vi "源强计算.vi"() -> ()   [LabVIEW 2020]
uses:
  <vilib>/Analysis/6fits.llb/Curve Fitting Criteria.ctl
  <vilib>/Utility/inputDevices.llb/mouseAcquire.vi
  <vilib>/gmath/NumericalOptimization/Nonlinear Curve Fit LM.vi
  <vilib>/gmath/NI_Gmath.lvlib
  <vilib>/Analysis/NI_AALPro.lvlib
panel:
  in  "本底迭代步长":dbl[](array[numeric])=[0.0, 0.0, 0.0]
  in  "曲线显隐":bool[](array[boolean])
  in  "选项卡控件":enum32{"直线拟合(两参)", "混合多项式(三参)", "广指拟合(三参) "}(tab)
  in  "parameter bounds":T1={"slope min"=-inf, "slope max"=inf, "intercept min"=-inf, "intercept max"=inf} caption="参数界限"
  in  "初始参数":dbl[](array[numeric])
  in  "参数界限":T2={"amp min"=-inf, "amp max"=inf, "damping min"=-inf, "damping max"=inf, "offset min"=-inf, "offset max"=inf}
  in  "本底值":dbl[](array[numeric])=[0.0, 0.0, 0.0]
  out "两参法残差":dbl[](array[numeric])
  out "通量拟合源强":dbl[](array[numeric])
  out "两参法源强":dbl[](array[numeric])
  out "两参法反应性":dbl[](array[numeric])
  out "通量拟合残差":dbl[](array[numeric])
  in  "曲线标尺":bool[](array[boolean])
  in  "开始计算":bool
  in  "重选文件":bool
  in  "退出程序":bool
  out "提示信息":string
  out "filepath":path caption="数据文件路径和名称"
  out "数据采集起止时间":string
  out "DataGraph":dbl[][](graph)
  out "中间标位置":i32
  out "左选标位置":i32
  out "右选标位置":i32
  # "y=aX + b"
  # "y = a*exp(b*x) + c"
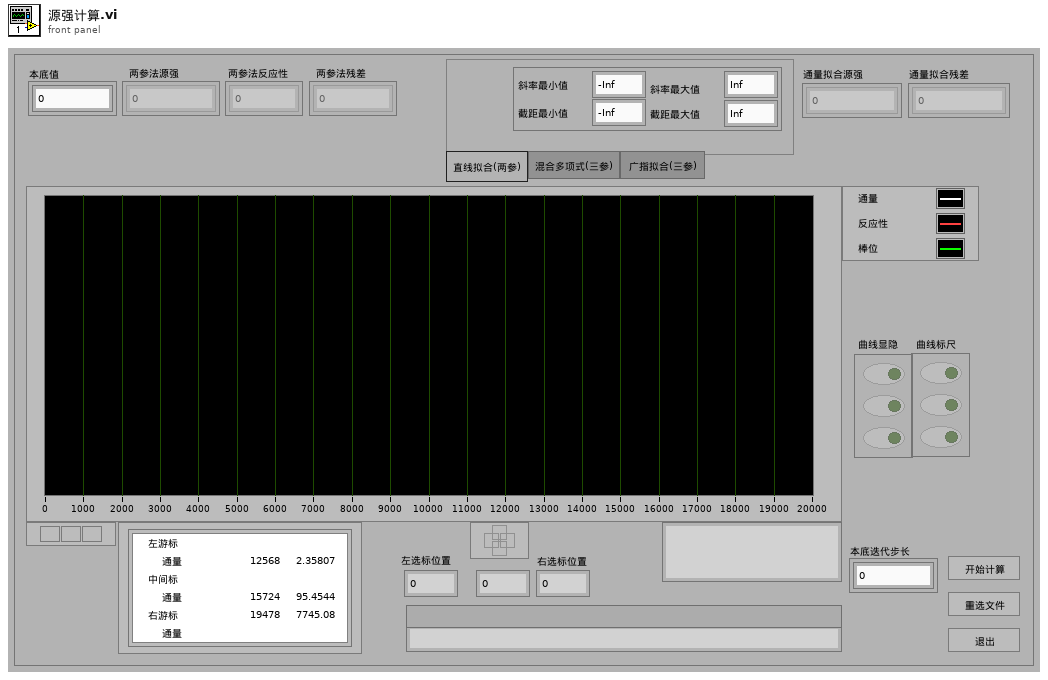
[diagram p1: front panel]
types:
  T1 = cluster{"slope min":dbl, "slope max":dbl, "intercept min":dbl, "intercept max":dbl}
  T2 = cluster{"amp min":dbl, "amp max":dbl, "damping min":dbl, "damping max":dbl, "offset min":dbl, "offset max":dbl}
  T3 = cluster{"button 1":bool, "button 2":bool, "button 3":bool, "button 4":bool}
  T4 = typedef "LVCursorListTypeDef.ctl" = cluster{"Name":string, "Color":u32, "Style":u8, "Point Style":u8, "Name Visible":bool, "Allow Drag":bool, "Cursor Mode":u32, "Plot":i32, "Index":i32, "Position":cluster{"X":dbl, "Y":dbl}, "X Scale":u32, "Y Scale":u32, "Watch Plots":i32[], "Watch All Plots":bool, "Plot Area":i32, "Label Offset":cluster{"X":dbl, "Y":dbl}}[]
  T5 = cluster{"Name":string, "Color":u32, "Style":u8, "Point Style":u8, "Name Visible":bool, "Allow Drag":bool, "Cursor Mode":u32, "Plot":i32, "Index":i32, "Position":cluster{"X":dbl, "Y":dbl}, "X Scale":u32, "Y Scale":u32, "Watch Plots":i32[], "Watch All Plots":bool, "Plot Area":i32, "Label Offset":cluster{"X":dbl, "Y":dbl}}
  T6 = typedef "NI_AALPro.lvlib/Curve Fitting Criteria.ctl" = u16
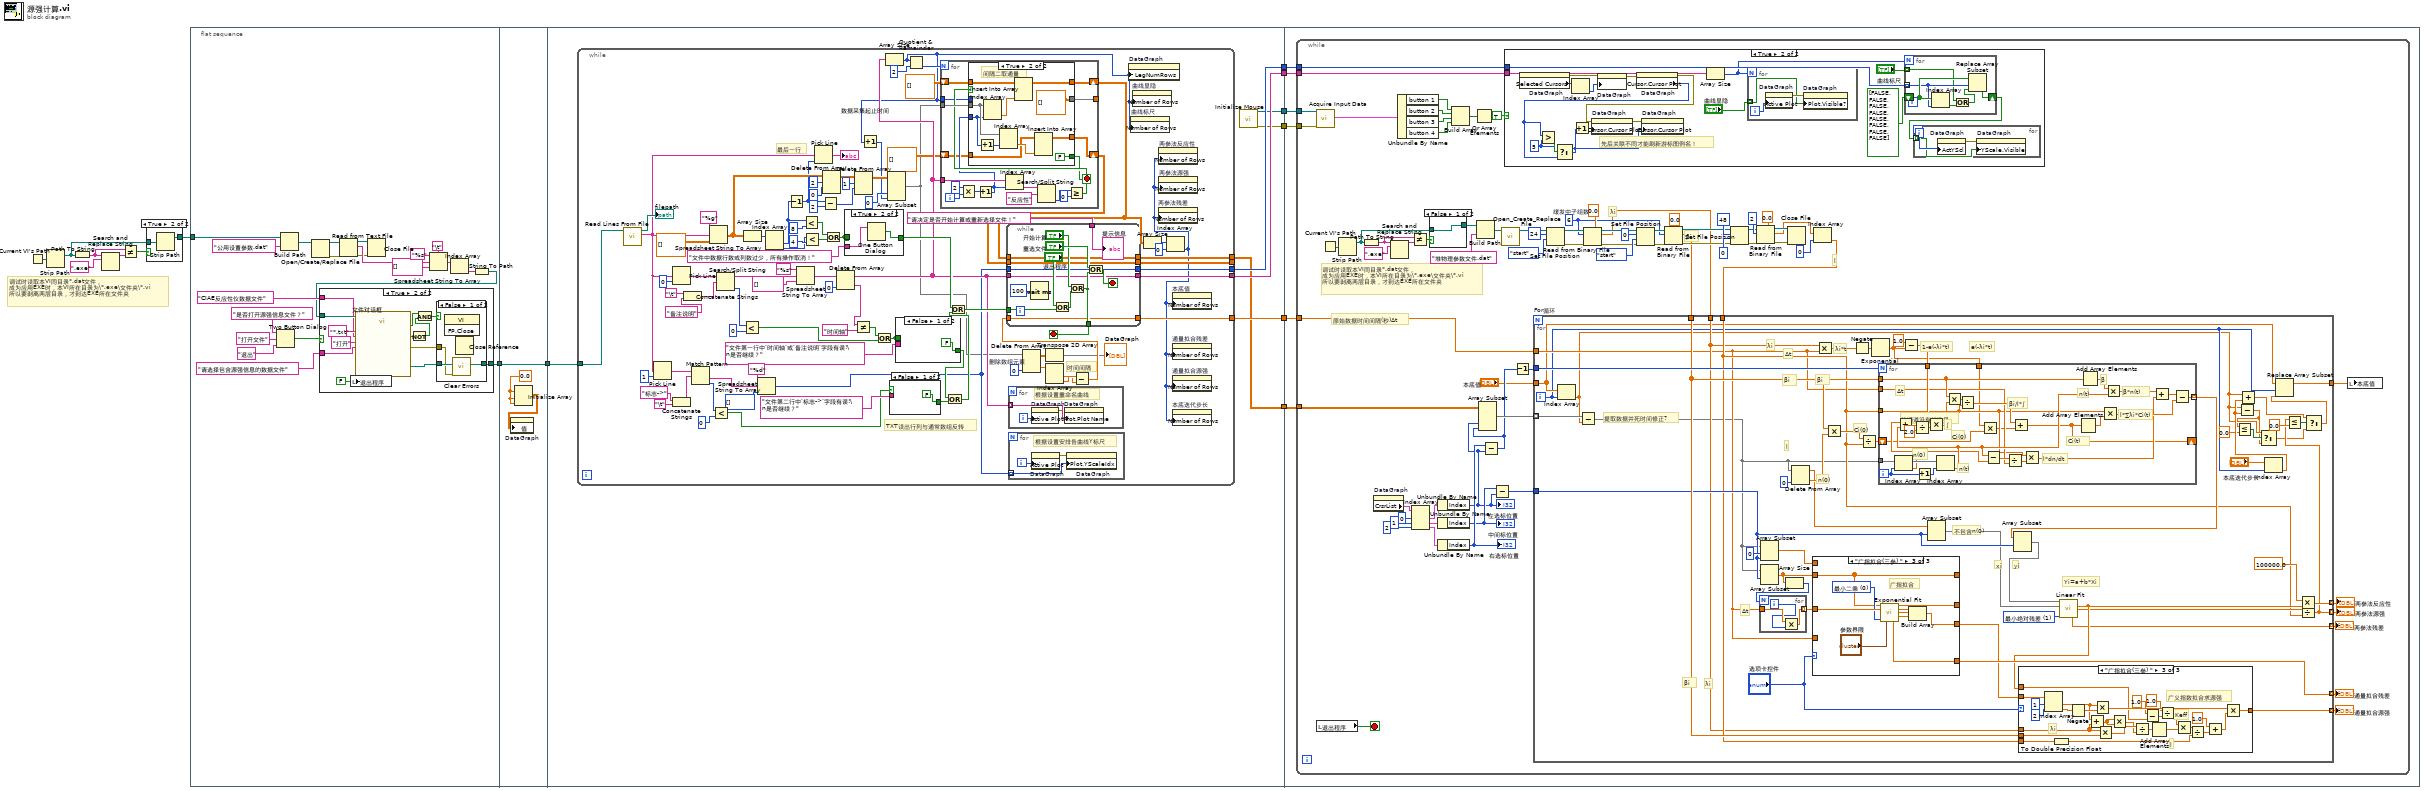
[diagram p0: block diagram]
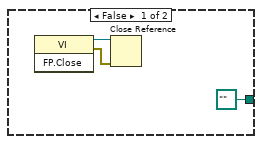
[diagram p3: hidden frame]
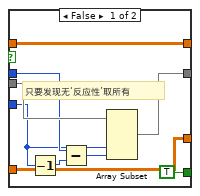
[diagram p5: hidden frame]
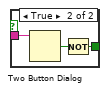
[diagram p6: hidden frame]
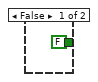
[diagram p7: hidden frame]
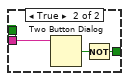
[diagram p8: hidden frame]
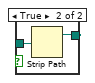
[diagram p10: hidden frame]
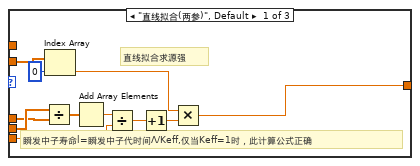
[diagram p11: hidden frame]
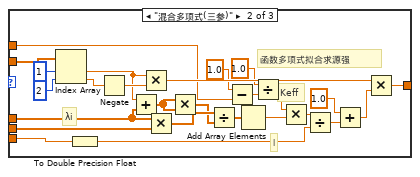
[diagram p12: hidden frame]
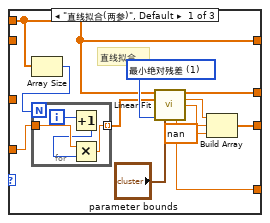
[diagram p13: hidden frame]
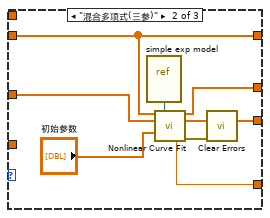
[diagram p14: hidden frame]
diagram:
  # "调试时读取本VI同目录*.dat文件，\n成为应用EXE时，本VI所在目录为\\*.exe\\文件夹\\*.vi\n所以要剥离两层目录，才到达EXE所在文件夹"
  n1 = Current VI's Path() -> (path=w4:path)
  n2 = Strip Path(path=w4) -> (stripped path=w9:path)  [unwired: 1 out]
  n3 = Path To String(path=w9) -> (string=w7:string)
  n4 = Search and Replace String(input string=w7, search string=".exe" ("搜索字符串")) -> (result string=w6:string)  [unwired: 6 in, 3 out]
  n5 = Not Equal?(x=w7, y=w6) -> (x != y?=w8:bool)
  n6 = case shown="True" w8 {
    tunnel: w9 -> [w16 w18]
    tunnel: [w16 w17] -> w3
    frame False {
    }
    frame True {
      n7 = Strip Path(path=w18) -> (stripped path=w17:path)  [unwired: 1 out]
    }
  }
  n8 = flat-sequence {
    tunnel: w3 -> [w20]
    tunnel: [w19] -> w2
    tunnel: w2 -> [w61]
    tunnel: [w61] -> w1
    tunnel: [w65] -> w15
    tunnel: [w70] -> w14
    tunnel: [w69] -> w13
    tunnel: [w68] -> w12
    tunnel: [w67] -> w11
    tunnel: [w66] -> w10
    tunnel: w1 -> [w64]
    tunnel: w15 -> [w233]
    tunnel: w14 -> [w232]
    tunnel: w13 -> [w231]
    tunnel: w12 -> [w230]
    tunnel: w11 -> [w228]
    tunnel: w10 -> [w229]
    frame #0 {
      n9 = Two Button Dialog(message="是否打开源强信息文件？", 1:"退出" ("message"), 2:"打开文件" ("message")) -> (T button?=w36:bool)
      n10 = Build Path(base path=w20, name or relative path="公用设置参数.dat") -> (appended path=w26:path)
      n11 = Open/Create/Replace File(file path (use dialog)=w26) -> (refnum out=w29:refnum<file>, error out=w30:errorcluster)  [unwired: 5 in, 1 out]
      n12 = Read from Text File(file (use dialog)=w29, error in=w30) -> (refnum out=w28:refnum<file>, text=w34:string, error out=w27:errorcluster)  [unwired: 1 in, 2 out]
      n13 = Close File(refnum=w28, error in=w27) -> ()  [unwired: 2 out]
      n14 = Spreadsheet String To Array(delimiter (Tab)="\t", format string="%s", spreadsheet string=w34, array type (2D Dbl)=string[] [] ("添加的数组")) -> (array=w35:string[])
      n15 = Index Array(array=w35) -> (element=w24:string)  [unwired: 1 in]
      n16 = String To Path(string=w24) -> (path=w37:path)
      n17 = case shown="True" w36 {
        tunnel: w37 -> [_ w55]
        tunnel: "请选择包含源强信息的数据文件" ("prompt") -> [_ w51]
        tunnel: "CIAE反应性仪数据文件" ("pattern label") -> [_ w50]
        tunnel: [path "" ("selected path") w48] -> w19
        frame False {
          n18 = invoke class="VI" method="FP.Close"() -> (reference out=w41:refnum<vi>, error out=w40:errorcluster)  [unwired: 3 in, 1 out]
          n19 = Close Reference(reference=w41, error in (no error)=w40) -> ()  [unwired: 1 out]
        }
        frame True {
          n20 = local write "退出程序"(FALSE ("退出程序")) -> ()
          n21 = call "文件对话框"("start path"=w55, "prompt"=w51, "button label"="打开", "pattern (all files)"="*.txt", "pattern label"=w50) -> ("selected path"=w49:path, "exists"=w46:bool, "cancelled"=w47:bool, "error out"=w43:errorcluster)  [unwired: 7 in]
          n22 = Not(x=w47) -> (.not. x?=w45:bool)
          n23 = And(x=w46, y=w45) -> (x .and. y?=w44:bool)
          n24 = case shown="False" w44 {
            tunnel: w49 -> [w59 w60]
            tunnel: [w59 w60] -> w48
            tunnel: w43 -> [w58 _]
            frame False {
              n25 = invoke class="VI" method="FP.Close"() -> (reference out=w57:refnum<vi>, error out=w56:errorcluster)  [unwired: 3 in, 1 out]
              n26 = call <vilib>:"Clear Errors.vi"("error in (no error)"=w58) -> ()  [unwired: 5 in, 2 out]
              n27 = Close Reference(reference=w57, error in (no error)=w56) -> ()  [unwired: 1 out]
            }
            frame True {
            }
          }
        }
      }
    }
    frame #1 {
      w63 = sgl 0.0
      n28 = Initialize Array(w63, w63, w63) -> (w62:sgl[][])
      n29 = property on="DataGraph" class="WFGraph (strict)"("值"=w62) -> ()  [unwired: 2 in, 2 out]
    }
    frame #2 {
      n30 = while {
        tunnel: [w100] -> _
        tunnel: [w151] -> w69
        tunnel: [w98] -> w68
        tunnel: [w99] -> w65
        tunnel: [w87] -> w70
        tunnel: w64 -> [w73]
        stop <- w157 stop-if-true
        # "时间间隔"
        # "TXT读出行列与通常数组反转"
        # "最后一行"
        n31 = call <vilib>:"Read Lines From File.vi"("file path (dialog if empty)"=w73) -> ("new file path (Not A Path if cancelled)"=→"filepath":path, "line string"=w105:string)  [unwired: 5 in, 2 out]
        n32 = Pick Line(multi-line string=w105, line index=1 ("行索引")) -> (output string=w130:string)  [unwired: 1 in]
        n33 = Pick Line(multi-line string=w105, line index=0 ("行索引")) -> (output string=w149:string)  [unwired: 1 in]
        n34 = Concatenate Strings("标志->" ("搜索字符串/字符(-)"), "\t") -> (w127:string)
        n35 = Concatenate Strings("\t", "备注说明" ("搜索字符串/字符(-)")) -> (w109:string)
        n36 = Match Pattern(string=w130, regular expression=w127) -> (after substring=w124:string, offset past match=w118:i32)  [unwired: 1 in, 2 out]
        n37 = Spreadsheet String To Array ("电子表格字符串至数组转换")(format string="%g" ("format (%.3f)"), spreadsheet string=w105, array type (2D Dbl)=dbl[][] [] ("type (empty)")) -> (array=w111:dbl[][])  [unwired: 1 in]
        n38 = Less?(x=w118, y=0) -> (x < y?=w117:bool)
        n39 = Search/Split String(string=w149, search string/char (-)=w109) -> (substring before match=w148:string, offset of match=w147:i32)  [unwired: 1 in, 1 out]
        n40 = Less?(x=w147, y=0) -> (x < y?=w144:bool)
        n41 = Array Size(array=w111) -> (size(s)=w158:i32[])
        n42 = Spreadsheet String To Array ("电子表格字符串至数组转换")(format string="%d" ("format (%.3f)"), spreadsheet string=w124, array type (2D Dbl)=i32[] [] ("添加的数组")) -> (array=w96:i32[])  [unwired: 1 in]
        n43 = Index Array(array=w158) -> (element #1=w104:i32, element #2=w138:i32)  [unwired: 2 in]
        n44 = Decrement(x=w104) -> (x-1=w76:i32)
        n45 = Spreadsheet String To Array ("电子表格字符串至数组转换")(format string="%s" ("format (%.3f)"), spreadsheet string=w148, array type (2D Dbl)=string[] [] ("添加的数组")) -> (array=w116:string[])  [unwired: 1 in]
        n46 = Less?(x=w104, y=8) -> (x < y?=w136:bool)
        n47 = Less?(x=w138, y=4) -> (x < y?=w135:bool)
        n48 = Pick Line ("选行并添加至字符串")(multi-line string=w105, line index=w76) -> (output string=→"数据采集起止时间":string)  [unwired: 1 in]
        n49 = Subtract(x=w76, y=2) -> (x-y=w75:i32)
        n50 = Delete From Array(array=w111, length=2 ("长度"), index (row)=0 ("索引")) -> (array with subset deleted=w110:dbl[][])  [unwired: 1 in, 1 out]
        n51 = Or(x=w136, y=w135) -> (x .or. y?=w137:bool)
        n52 = Delete From Array(array=w116, index=0 ("索引")) -> (deleted portion=w84:string, array with subset deleted=w97:string[])  [unwired: 1 in]
        n53 = case shown="True" w137 {
          tunnel: w137 -> [_ _]
          tunnel: [FALSE w208] -> w132
          tunnel: "文件中数据行数或列数过少，所有操作取消！" ("y") -> [_ w209]
          frame False {
          }
          frame True {
            n54 = One Button Dialog(message=w209) -> (true=w208:bool)  [unwired: 1 in]
          }
        }
        n55 = Not Equal?(x=w84, y="时间轴") -> (x != y?=w143:bool)
        n56 = Delete From Array(array=w110, length=1 ("长度"), index (row)=w75) -> (array with subset deleted=w83:dbl[][])  [unwired: 1 in, 1 out]
        n57 = Or(x=w143, y=w144) -> (x .or. y?=w142:bool)
        n58 = Array Size(array=w97) -> (size(s)=w72:i32)
        n59 = Increment(x=w72) -> (x+1=w80:i32)
        n60 = Array Subset ("数组子集")(array=w83, index (col)=0 ("索引"), length (col)=w80) -> (w82:dbl[][])  [unwired: 2 in]
        n61 = case shown="False" w117 {
          tunnel: "文件第二行中‘标志->’字段有误!\n是否继续？" ("y") -> [_ w206]
          tunnel: [FALSE w204] -> w122
          frame False {
          }
          frame True {
            n62 = Two Button Dialog(message=w206) -> (T button?=w205:bool)  [unwired: 2 in]
            n63 = Not(x=w205) -> (.not. x?=w204:bool)
          }
        }
        n64 = case shown="False" w142 {
          tunnel: w142 -> [_ _]
          tunnel: "文件第一行中‘时间轴’或‘备注说明’字段有误!\n是否继续？" ("y") -> [_ w213]
          tunnel: [FALSE w211] -> w121
          frame False {
          }
          frame True {
            n65 = Two Button Dialog(message=w213) -> (T button?=w212:bool)  [unwired: 2 in]
            n66 = Not(x=w212) -> (.not. x?=w211:bool)
          }
        }
        n67 = Quotient & Remainder(x=w72, y=2) -> (floor(x/y)=w101:i32)  [unwired: 1 out]
        n68 = for {
          N: w101 -> [_]
          tunnel: w82 -> [w175]
          tunnel: w97 -> [w182]
          shift-right: [w173] -> w77
          shift-left: dbl[][] [] ("type (empty)") -> [w174]
          tunnel: w72 -> [w169]
          tunnel: [w168] -> _
          shift-right: [w165] -> w92
          shift-left: dbl[][] [] ("type (empty)") -> [w166]
          i -> [w181]
          stop <- w170 stop-if-true
          n69 = Multiply(x=2, y=w181) -> (x*y=w167:i32)
          n70 = Increment(x=w167) -> (x+1=w171:i32)
          n71 = Index Array(array=w182, index=w171) -> (element=w179:string)
          n72 = Search/Split String(string=w179, search string/char (-)="反应性" ("搜索字符串/字符(-)")) -> (offset of match=w177:i32)  [unwired: 1 in, 2 out]
          n73 = Greater Or Equal?(x=w177, y=0) -> (x >= y?=w172:bool)
          n74 = case shown="True" w172 {
            tunnel: w175 -> [w189 w197]
            tunnel: w174 -> [w191 w202]
            tunnel: [w191 w200] -> w173
            tunnel: w171 -> [w184 w192]
            tunnel: [TRUE FALSE] -> w170
            tunnel: w169 -> [w188 _]
            tunnel: [w185 dbl[][] [] ("type (empty)")] -> w168
            tunnel: w166 -> [w183 w195]
            tunnel: [w183 w194] -> w165
            frame False {
              # "只要发现无‘反应性’取所有"
              n75 = Decrement(x=w184) -> (x-1=w186:i32)
              n76 = Subtract(x=w188, y=w186) -> (x-y=w187:i32)
              n77 = Array Subset(array=w189, index (col)=w184, length (col)=w187) -> (w185:dbl[][])  [unwired: 2 in]
            }
            frame True {
              # "间隔二取通量"
              n78 = Increment(x=w192) -> (x+1=w193:i32)
              n79 = Index Array(array=w197, index (col)=w192) -> (element=w201:dbl[])  [unwired: 1 in]
              n80 = Index Array(array=w197, index (col)=w193) -> (element=w196:dbl[])  [unwired: 1 in]
              n81 = Insert Into Array(array=w202, new element=w201) -> (w200:dbl[][])  [unwired: 2 in]
              n82 = Insert Into Array(array=w195, new element=w196) -> (w194:dbl[][])  [unwired: 2 in]
            }
          }
        }
        n83 = Or(x=w121, y=w122) -> (x .or. y?=w120:bool)
        n84 = Or(x=w132, y=w120) -> (x .or. y?=w133:bool)
        n85 = for {
          tunnel: w97 -> [w163] mode=indexing
          i -> [w164]
          # "根据设置重命名曲线"
          n86 = property on="DataGraph" class="WFGraph (strict)"("Active Plot"=w164) -> (error out=w162:errorcluster)  [unwired: 2 in, 1 out]
          n87 = property on="DataGraph" class="WFGraph (strict)"(error in=w162, "Plot.Plot Name"=w163) -> ()  [unwired: 1 in, 2 out]
        }
        n88 = for {
          tunnel: w96 -> [w159] mode=indexing
          i -> [w161]
          # "根据设置安排各曲线Y标尺"
          n89 = property on="DataGraph" class="WFGraph (strict)"("Active Plot"=w161) -> (error out=w160:errorcluster)  [unwired: 2 in, 1 out]
          n90 = property on="DataGraph" class="WFGraph (strict)"(error in=w160, "Plot.YScaleIdx"=w159) -> ()  [unwired: 1 in, 2 out]
        }
        n91 = Delete From Array "删除数组元素"(array=w82, index (col)=0 ("禁用的索引 (列)")) -> (deleted portion=w91:dbl[], array with subset deleted=w95:dbl[][])  [unwired: 2 in]
        n92 = Transpose 2D Array(2D array=w95) -> (transposed array=→"DataGraph":dbl[][])
        n93 = Index Array(array=w91) -> (element #1=w89:dbl, element #2=w90:dbl)  [unwired: 2 in]
        n94 = Subtract(x=w90, y=w89) -> (x-y=w88:dbl)
        n95 = while {
          tunnel: [w218] -> w100
          tunnel: [w216] -> w151
          tunnel: w92 -> [w218]
          tunnel: w97 -> [w216]
          tunnel: [w225] -> w157
          tunnel: w133 -> [w221]
          tunnel: w77 -> [w219]
          tunnel: [w219] -> w99
          tunnel: w96 -> [w217]
          tunnel: [w217] -> w98
          tunnel: w88 -> [w215]
          tunnel: [w215] -> w87
          tunnel: "请决定是否开始计算或重新选择文件！" ("提示信息") -> [w214]
          stop <- w224 stop-if-true
          n96 = Wait (ms)(milliseconds to wait=u32 100 ("等待时间（毫秒）")) -> ()  [unwired: 1 out]
          n97 = Or(x="退出程序", y=w221) -> (x .or. y?=w222:bool)
          n98 = Or(x="开始计算", y=w222) -> (x .or. y?=w225:bool)
          n99 = Or(x="重选文件", y=w225) -> (x .or. y?=w224:bool)
          "提示信息" <- w214
        }
        n100 = property on="DataGraph" class="WFGraph (strict)"("LegNumRows"=w72) -> ()  [unwired: 2 in, 2 out]
        n101 = property on="曲线标尺" class="Arr (strict)"("Number of Rows"=w72) -> ()  [unwired: 2 in, 2 out]
        n102 = property on="曲线显隐" class="Arr (strict)"("Number of Rows"=w72) -> ()  [unwired: 2 in, 2 out]
        n103 = Array Size(array=w77) -> (size(s)=w78:i32[])
        n104 = Index Array(array=w78, index=0 ("索引")) -> (element=w71:i32)
        n105 = property on="两参法残差" class="Arr (strict)"("Number of Rows"=w71) -> ()  [unwired: 2 in, 2 out]
        n106 = property on="两参法反应性" class="Arr (strict)"("Number of Rows"=w71) -> ()  [unwired: 2 in, 2 out]
        n107 = property on="两参法源强" class="Arr (strict)"("Number of Rows"=w71) -> ()  [unwired: 2 in, 2 out]
        n108 = property on="本底值" class="Arr (strict)"("Number of Rows"=w71) -> ()  [unwired: 2 in, 2 out]
        n109 = property on="通量拟合残差" class="Arr (strict)"("Number of Rows"=w71) -> ()  [unwired: 2 in, 2 out]
        n110 = property on="通量拟合源强" class="Arr (strict)"("Number of Rows"=w71) -> ()  [unwired: 2 in, 2 out]
        n111 = property on="本底迭代步长" class="Arr (strict)"("Number of Rows"=w71) -> ()  [unwired: 2 in, 2 out]
      }
      n112 = call <vilib>:"Initialize Mouse.vi"() -> ("error out"=w66:errorcluster, "device ID"=w67:refnum<k1>)  [unwired: 1 in, 9 out]
    }
    frame #3 {
      n113 = while {
        tunnel: w233 -> [w264]
        tunnel: w232 -> [w243]
        tunnel: w231 -> [w277]
        tunnel: w230 -> [w278]
        tunnel: w228 -> [w270]
        tunnel: w229 -> [w269]
        stop <- w268 stop-if-true
        w288 = 6  # 缓发中子组数
        # "λi"
        # "l"
        # "调试时读取本VI同目录*.dat文件，\n成为应用EXE时，本VI所在目录为\\*.exe\\文件夹\\*.vi\n所以要剥离两层目录，才到达EXE所在文件夹"
        # "原始数据时间间隔(秒)Δt"
        # "βi"
        n114 = call-poly <vilib>:"Acquire Input Data.vi"("device ID"=w270, "error in (no error)"=w269) -> ("button info"=w276:T3)  [unwired: 1 in, 16 out]
        n115 = local read "退出程序"() -> (w268:bool)
        n116 = Current VI's Path() -> (path=w285:path)
        n117 = Strip Path(path=w285) -> (stripped path=w280:path)  [unwired: 1 out]
        n118 = Path To String(path=w280) -> (string=w282:string)
        n119 = property on="DataGraph" class="WFGraph (strict)"() -> ("CrsrList"=w294:T4)  [unwired: 2 in, 2 out]
        n120 = Search and Replace String(input string=w282, search string=".exe" ("搜索字符串")) -> (result string=w283:string)  [unwired: 6 in, 3 out]
        n121 = Unbundle By Name(w276) -> ("button 1"=w275:bool, "button 2"=w274:bool, "button 3"=w273:bool, "button 4"=w272:bool)
        n122 = Not Equal?(x=w282, y=w283) -> (x != y?=w281:bool)
        n123 = Index Array(array=w294, index #1=0 ("index"), index #2=1 ("index"), index #3=2 ("索引")) -> (element #1=w292:T5, element #2=w290:T5, element #3=w241:T5)
        n124 = case shown="False" w281 {
          tunnel: w280 -> [w337 w338]
          tunnel: [w337 w339] -> w279
          frame False {
          }
          frame True {
            n125 = Strip Path(path=w338) -> (stripped path=w339:path)  [unwired: 1 out]
          }
        }
        n126 = Unbundle By Name(w292) -> ("Index"=w238:i32)
        "左选标位置" <- w238
        n127 = Unbundle By Name(w290) -> ("Index"=w239:i32)
        "中间标位置" <- w239
        n128 = Unbundle By Name(w241) -> ("Index"=w240:i32)
        "右选标位置" <- w240
        n129 = Build Array(w275, w274, w273, w272) -> (w271:bool[])
        n130 = Or Array Elements(Boolean array=w271) -> ()  [unwired: 1 out]
        n131 = Build Path(base path=w279, name or relative path="堆物理参数文件.dat" ("string")) -> (appended path=w289:path)
        n132 = Subtract(x=w240, y=w238) -> (x-y=w244:i32)
        n133 = Array Subset(array=w264, index (col)=w238, length (col)=w244) -> (w263:dbl[][])  [unwired: 2 in]
        n134 = Subtract(x=w239, y=w238) -> (x-y=w237:i32)
        n135 = call <vilib>:"Open_Create_Replace File.vi"("file path"=w289) -> ("refnum"=w287:refnum<file>)  [unwired: 7 in, 3 out]
        n136 = case shown="True" TRUE {
          tunnel: w277 -> [_ w313]
          tunnel: w278 -> [_ w312]
          frame False {
          }
          frame True {
            w318 = 5 ("y")
            # "先后关联不同才能刷新游标图例名！"
            n137 = property on="DataGraph" class="WFGraph (strict)"() -> (error out=w322:errorcluster, "Selected Cursors"=w324:u32[])  [unwired: 2 in, 1 out]
            n138 = Index Array(array=w324) -> (element=w323:u32)  [unwired: 1 in]
            n139 = property on="DataGraph" class="WFGraph (strict)"(error in=w322, "Active Cursor"=w323) -> (error out=w321:errorcluster)  [unwired: 1 in, 1 out]
            n140 = property on="DataGraph" class="WFGraph (strict)"(error in=w321) -> (error out=w315:errorcluster, "Cursor.Cursor Plot"=w319:i32)  [unwired: 1 in, 1 out]
            n141 = Greater?(x=w319, y=w318) -> (0:w320:bool)
            n142 = Select(t=w318, s=w320, f=w319) -> (s? t:f=w314:i32)
            n143 = Increment(x=w314) -> (x+1=w316:i32)
            n144 = property on="DataGraph" class="WFGraph (strict)"(error in=w315, "Cursor.Cursor Plot"=w316) -> (error out=w317:errorcluster)  [unwired: 1 in, 1 out]
            n145 = property on="DataGraph" class="WFGraph (strict)"(error in=w317, "Cursor.Cursor Plot"=w314) -> ()  [unwired: 1 in, 2 out]
            n146 = Array Size(array=w313) -> (size(s)=w310:i32)
            n147 = for {
              N: w310 -> [_]
              tunnel: "曲线显隐" -> [w328] mode=indexing
              i -> [w329]
              n148 = property on="DataGraph" class="WFGraph (strict)"("Active Plot"=w329) -> (error out=w330:errorcluster)  [unwired: 2 in, 1 out]
              n149 = property on="DataGraph" class="WFGraph (strict)"(error in=w330, "Plot.Visible?"=w328) -> ()  [unwired: 1 in, 2 out]
            }
            n150 = for {
              N: w310 -> [_]
              tunnel: w312 -> [w335] mode=indexing
              tunnel: "曲线标尺" -> [w333] mode=indexing
              shift-right: [w331] -> w308
              shift-left: bool[] [FALSE, FALSE, FALSE, FALSE, FALSE, FALSE, FALSE, FALSE] ("曲线标尺") -> [w336]
              n151 = Index Array(array=w336, index=w335) -> (element=w334:bool)
              n152 = Or(x=w333, y=w334) -> (x .or. y?=w332:bool)
              n153 = Replace Array Subset(array=w336, new element=w332, index=w335) -> (w331:bool[])
            }
            n154 = for {
              tunnel: w308 -> [w326] mode=indexing
              i -> [w327]
              n155 = property on="DataGraph" class="WFGraph (strict)"("ActYScl"=w327) -> (error out=w325:errorcluster)  [unwired: 2 in, 1 out]
              n156 = property on="DataGraph" class="WFGraph (strict)"(error in=w325, "YScale.Visible"=w326) -> ()  [unwired: 1 in, 2 out]
            }
          }
        }
        n157 = Decrement(x=w244) -> (x-1=w265:i32)
        n158 = Set File Position(offset (in bytes) (0)=24 ("pos offset (0)"), refnum=w287, from (0:start)=enum16{"start", "end", "current"}."start" ("pos mode (0:2)")) -> (refnum out=w299:refnum<file>, error out=w302:errorcluster)  [unwired: 1 in]
        n159 = Read from Binary File(5:sgl 0.0, 8:w302, 10:w288, 11:w299) -> (0:w296:errorcluster, 2:w245:sgl[], 3:w297:refnum<file>)  [unwired: 2 in, 1 out]
        n160 = Set File Position(offset (in bytes) (0)=0, refnum=w297, from (0:start)=enum16{"start", "end", "current"}."start" ("pos mode (0:2)"), error in=w296) -> (refnum out=w301:refnum<file>, error out=w300:errorcluster)
        n161 = Read from Binary File(5:sgl 0.0, 8:w300, 10:w288, 11:w301) -> (0:w253:errorcluster, 2:w246:sgl[], 3:w254:refnum<file>)  [unwired: 2 in, 1 out]
        n162 = Set File Position(offset (in bytes) (0)=48, refnum=w254, from (0:start)=0, error in=w253) -> (refnum out=w256:refnum<file>, error out=w255:errorcluster)
        n163 = Read from Binary File(5:sgl 0.0, 8:w255, 10:2, 11:w256) -> (0:w251:errorcluster, 2:w250:sgl[], 3:w252:refnum<file>)  [unwired: 2 in, 1 out]
        n164 = Close File(refnum=w252, error in=w251) -> ()  [unwired: 2 out]
        n165 = Index Array(array=w250, index=0 ("索引")) -> (element=w248:sgl)
        n166 = for "For循环" {
          tunnel: w263 -> [w361] mode=indexing
          tunnel: w243 -> [w363]
          tunnel: w265 -> [w390]
          tunnel: [w388] -> w266 mode=indexing
          tunnel: [w387] -> w262 mode=indexing
          tunnel: [w350] -> w261 mode=indexing
          tunnel: w246 -> [w380]
          tunnel: w245 -> [w366]
          tunnel: w248 -> [w370]
          tunnel: [w384] -> w247 mode=indexing
          tunnel: w237 -> [w373]
          tunnel: [w362] -> w236 mode=indexing
          tunnel: "本底值" -> [w354]
          tunnel: [w353] -> w234
          i -> [w348]
          w389 = T6 1 items=["最小二乘", "最小绝对残差", "Bisquare"] ("method")
          # "βi"
          # "Δt"
          # "Δt"
          # "λi"
          # "e(-λi*t)"
          # "1-e(-λi*t)"
          # "λi*t"
          # "λi"
          # "βi"
          # "不包含n(0)"
          # "Yi=a+b*Xi"
          # "l"
          # "βi"
          # "yi"
          # "n(0)"
          # "提取数据并死时间修正?"
          # "xi"
          # "Ci(0)"
          # "该通道没有被选择"
          n167 = Index Array(array=w354, index=w348) -> (element=w342:dbl)
          n168 = Subtract(x=w361, y=w342) -> (x-y=w360:dbl[])
          n169 = Array Subset(array=w360, index=w373) -> (w359:dbl[])  [unwired: 1 in]
          n170 = Array Subset(array=w360, index=0 ("索引"), length=w373) -> (w372:dbl[])
          n171 = Array Size(array=w359) -> (size(s)=w386:i32)
          n172 = for {
            N: w386 -> [_]
            tunnel: [w490] -> w385 mode=indexing
            tunnel: w363 -> [w489]
            i -> [w488]
            n173 = Multiply(x=w489, y=w488) -> (x*y=w490:dbl)
          }
          n174 = Delete From Array(array=w360, index=0 ("长度")) -> (deleted portion=w376:dbl, array with subset deleted=w375:dbl[])  [unwired: 1 in]
          n175 = case shown="\"广指拟合(三参) \"" "选项卡控件" {
            tunnel: [w465 w475 w482] -> w388
            tunnel: w359 -> [_ w471 w479]
            tunnel: w385 -> [_ w474 w484]
            tunnel: [w464 w473 w483] -> w356
            tunnel: w372 -> [w456 _ _]
            tunnel: w363 -> [w457 _ _]
            tunnel: [w455 w472 w480] -> _
            tunnel: [w456 w471 w479] -> _
            frame "直线拟合(两参)", Default {
              w460 = T6 1 items=["最小二乘", "最小绝对残差", "Bisquare"] ("method")
              # "直线拟合"
              n176 = Array Size(array=w456) -> (size(s)=w458:i32)
              n177 = for {
                N: w458 -> [_]
                tunnel: [w469] -> w459 mode=indexing
                tunnel: w457 -> [w468]
                i -> [w467]
                n178 = Increment(x=w467) -> (x+1=w466:i32)
                n179 = Multiply(x=w468, y=w466) -> (x*y=w469:dbl)
              }
              n180 = call <vilib>:"Linear Fit.vi"("Y"=w456, "X"=w459, "method"=w460, "parameter bounds"="parameter bounds") -> ("Best Linear Fit"=w455:dbl[], "slope"=w463:dbl, "intercept"=w462:dbl, "residue"=w465:dbl)  [unwired: 7 in, 1 out]
              n181 = Build Array(w463, w462, nan ("元素")) -> (w464:dbl[])
            }
            frame "混合多项式(三参)" {
              n182 = vi-ref "simple exp model.vi"() -> (w477:refnum<vi>)
              n183 = call-poly <vilib>:"Nonlinear Curve Fit.vi"("Y"=w471, "f(x,a)"=w477, "X"=w474, "initial parameters"="初始参数") -> ("best nonlinear fit"=w472:dbl[], "best fit parameters"=w473:dbl[], "residue"=w475:dbl, "error out"=w476:errorcluster)  [unwired: 6 in, 2 out]
              n184 = call <vilib>:"Clear Errors.vi"("error in (no error)"=w476) -> ()  [unwired: 5 in, 2 out]
            }
            frame "广指拟合(三参) " {
              w481 = T6 0 items=["最小二乘", "最小绝对残差", "Bisquare"] ("method")
              # "广指拟合"
              n185 = call <vilib>:"Exponential Fit.vi"("Y"=w479, "X"=w484, "method"=w481, "parameter bounds"="参数界限") -> ("Best Exponential Fit"=w480:dbl[], "amplitude"=w487:dbl, "damping"=w486:dbl, "offset"=w485:dbl, "residue"=w482:dbl)  [unwired: 6 in, 1 out]
              n186 = Build Array(w487, w486, w485) -> (w483:dbl[])
            }
          }
          n187 = Multiply(x=w366, y=w363) -> (x*y=w367:dbl[])
          n188 = Multiply(x=w380, y=w376) -> (x*y=w379:dbl[])
          n189 = Negate(x=w367) -> (-x=w368:dbl[])
          n190 = Divide(x=w379, y=w370) -> (x/y=w382:dbl[])
          n191 = Exponential(1:w368) -> (0:w364:dbl[])
          n192 = Subtract(x=1.0, y=w364) -> (x-y=w365:dbl[])
          n193 = for {
            N: w390 -> [_]
            shift-right: [w491] -> _
            shift-left: w382 -> [w494]
            tunnel: w360 -> [w516]
            tunnel: w365 -> [w513]
            tunnel: w380 -> [w506]
            tunnel: w370 -> [w499]
            tunnel: [w505] -> w378 mode=indexing
            tunnel: w364 -> [w493]
            tunnel: w363 -> [w501]
            i -> [w518]
            # "Δt"
            # "l*dn/dt"
            # "n(t)"
            # "β"
            # "βi/l*∫"
            # "Ci(0)"
            # "∫"
            # "l*∑λi*Ci(t)"
            # "β*n(t)"
            # "n(t)"
            # "Ci(t)"
            # "n(0)"
            n194 = Index Array(array=w516, index=w518) -> (element=w503:dbl)
            n195 = Increment(x=w518) -> (x+1=w517:i32)
            n196 = Index Array(array=w516, index=w517) -> (element=w504:dbl)
            n197 = Add(x=w503, y=w504) -> (x+y=w515:dbl)
            n198 = Divide(x=w515, y=2.0) -> (x/y=w510:dbl)
            n199 = Multiply(x=w513, y=w510) -> (x*y=w495:dbl[])
            n200 = Multiply(x=w506, y=w495) -> (x*y=w512:dbl[])
            n201 = Divide(x=w512, y=w499) -> (x/y=w511:dbl[])
            n202 = Multiply(x=w493, y=w494) -> (x*y=w492:dbl[])
            n203 = Subtract(x=w504, y=w503) -> (x-y=w502:dbl)
            n204 = Divide(x=w502, y=w501) -> (x/y=w500:dbl)
            n205 = Add(x=w511, y=w492) -> (x+y=w491:dbl[])
            n206 = Multiply(x=w499, y=w500) -> (x*y=w496:dbl)
            n207 = Add Array Elements(numeric array=w491) -> (sum=w509:dbl)
            n208 = Add Array Elements(numeric array=w506) -> (sum=w507:sgl)
            n209 = Multiply(x=w499, y=w509) -> (x*y=w508:dbl)
            n210 = Multiply(x=w507, y=w504) -> (x*y=w497:dbl)
            n211 = Add(x=w497, y=w496) -> (x+y=w498:dbl)
            n212 = Subtract(x=w498, y=w508) -> (x-y=w505:dbl)
          }
          n213 = Array Subset(array=w375, index=w373) -> (w358:dbl[])  [unwired: 1 in]
          n214 = Array Subset(array=w378, index=w373) -> (w357:dbl[])  [unwired: 1 in]
          n215 = call <vilib>:"Linear Fit.vi"("Y"=w357, "X"=w358, "method"=w389) -> ("slope"=w383:dbl, "intercept"=w371:dbl, "residue"=w362:dbl)  [unwired: 8 in, 2 out]
          n216 = case shown="\"广指拟合(三参) \"" "选项卡控件" {
            tunnel: w356 -> [w392 w427 w431]
            tunnel: w380 -> [w401 w422 w429]
            tunnel: w366 -> [w400 w421 w430]
            tunnel: w370 -> [w397 w406 w428]
            tunnel: [w393 w403 w433] -> w384
            tunnel: w383 -> [_ w407 w432]
            frame "直线拟合(两参)", Default {
              # "瞬发中子寿命l=瞬发中子代时间Λ/Keff,仅当Keff=1时，此计算公式正确"
              # "直线拟合求源强"
              n217 = Divide(x=w401, y=w400) -> (x/y=w399:sgl[])
              n218 = Index Array(array=w392, index=0 ("索引")) -> (element=w391:dbl)
              n219 = Add Array Elements(numeric array=w399) -> (sum=w398:sgl)
              n220 = Divide(x=w398, y=w397) -> (x/y=w396:sgl)
              n221 = Increment(x=w396) -> (x+1=w394:sgl)
              n222 = Multiply(x=w391, y=w394) -> (x*y=w393:dbl)
            }
            frame "混合多项式(三参)" {
              # "Keff"
              # "l"
              # "λi"
              # "函数多项式拟合求源强"
              n223 = Index Array(array=w427, index #1=1 ("索引"), index #2=2 ("索引")) -> (element #1=w404:dbl, element #2=w424:dbl)
              n224 = To Double Precision Float(number=w406) -> (double precision float=w405:dbl)
              n225 = Negate(x=w424) -> (-x=w423:dbl)
              n226 = Add(x=w404, y=w421) -> (x+y=w420:dbl[])
              n227 = Multiply(x=w404, y=w423) -> (x*y=w414:dbl)
              n228 = Multiply(x=w421, y=w422) -> (x*y=w419:sgl[])
              n229 = Multiply(x=w420, y=w420) -> (x*y=w418:dbl[])
              n230 = Divide(x=w419, y=w418) -> (x/y=w417:dbl[])
              n231 = Subtract(x=1.0, y=w407) -> (x-y=w409:dbl)
              n232 = Add Array Elements(numeric array=w417) -> (sum=w412:dbl)
              n233 = Divide(x=1.0, y=w409) -> (x/y=w402:dbl)
              n234 = Multiply(x=w402, y=w412) -> (x*y=w411:dbl)
              n235 = Divide(x=w411, y=w405) -> (x/y=w416:dbl)
              n236 = Add(x=1.0, y=w416) -> (x+y=w413:dbl)
              n237 = Multiply(x=w414, y=w413) -> (x*y=w403:dbl)
            }
            frame "广指拟合(三参) " {
              # "Keff"
              # "l"
              # "λi"
              # "广义指数拟合求源强"
              n238 = Index Array(array=w431, index #1=1 ("索引"), index #2=2 ("索引")) -> (element #1=w435:dbl, element #2=w451:dbl)
              n239 = To Double Precision Float(number=w428) -> (double precision float=w436:dbl)
              n240 = Negate(x=w451) -> (-x=w450:dbl)
              n241 = Add(x=w435, y=w430) -> (x+y=w449:dbl[])
              n242 = Multiply(x=w435, y=w450) -> (x*y=w443:dbl)
              n243 = Multiply(x=w430, y=w429) -> (x*y=w448:sgl[])
              n244 = Multiply(x=w449, y=w449) -> (x*y=w447:dbl[])
              n245 = Divide(x=w448, y=w447) -> (x/y=w446:dbl[])
              n246 = Subtract(x=1.0, y=w432) -> (x-y=w438:dbl)
              n247 = Add Array Elements(numeric array=w446) -> (sum=w441:dbl)
              n248 = Divide(x=1.0, y=w438) -> (x/y=w434:dbl)
              n249 = Multiply(x=w434, y=w441) -> (x*y=w440:dbl)
              n250 = Divide(x=w440, y=w436) -> (x/y=w445:dbl)
              n251 = Add(x=1.0, y=w445) -> (x+y=w442:dbl)
              n252 = Multiply(x=w443, y=w442) -> (x*y=w433:dbl)
            }
          }
          n253 = Index Array(array="本底迭代步长", index=w348) -> (element=w347:dbl)
          n254 = Subtract(x=w342, y=w347) -> (x-y=w340:dbl)
          n255 = Less Or Equal?(x=w340, y=0.0) -> (x <= y?=w343:bool)
          n256 = Add(x=w342, y=w347) -> (x+y=w346:dbl)
          n257 = Select(t=w342, s=w343, f=w340) -> (s? t:f=w341:dbl)
          n258 = Multiply(x=sgl 100000.0 ("y"), y=w383) -> (x*y=w387:dbl)
          n259 = Divide(x=w371, y=w370) -> (x/y=w350:dbl)
          n260 = Less Or Equal?(x=w350, y=0.0) -> (x <= y?=w351:bool)
          n261 = Select(t=w346, s=w351, f=w341) -> (s? t:f=w345:dbl)
          n262 = Replace Array Subset(array=w354, new element=w345, index=w348) -> (w353:dbl[])
        }
        "通量拟合残差" <- w266
        "两参法反应性" <- w262
        "两参法源强" <- w261
        "通量拟合源强" <- w247
        "两参法残差" <- w236
        n263 = local write "本底值"(w234) -> ()
      }
    }
  }
